vi "Update Objective tree.vi"(7 "Visible Items:Column Headers Visible":bool, 8 "error in (no error)":errorcluster, 9 "Column Header Strings[]":string[](array[string]), 10 "Config cluster IN":T1, 11 "TreeControl in":refnum<vi>) -> (0 "error out":errorcluster)   [LabVIEW 2020]
uses:
  Typedefs/Calibration config.ctl
  Typedefs/Objective Config.ctl
  Typedefs/Prechirper Cal Config.ctl
  Typedefs/PreChirper constants.ctl
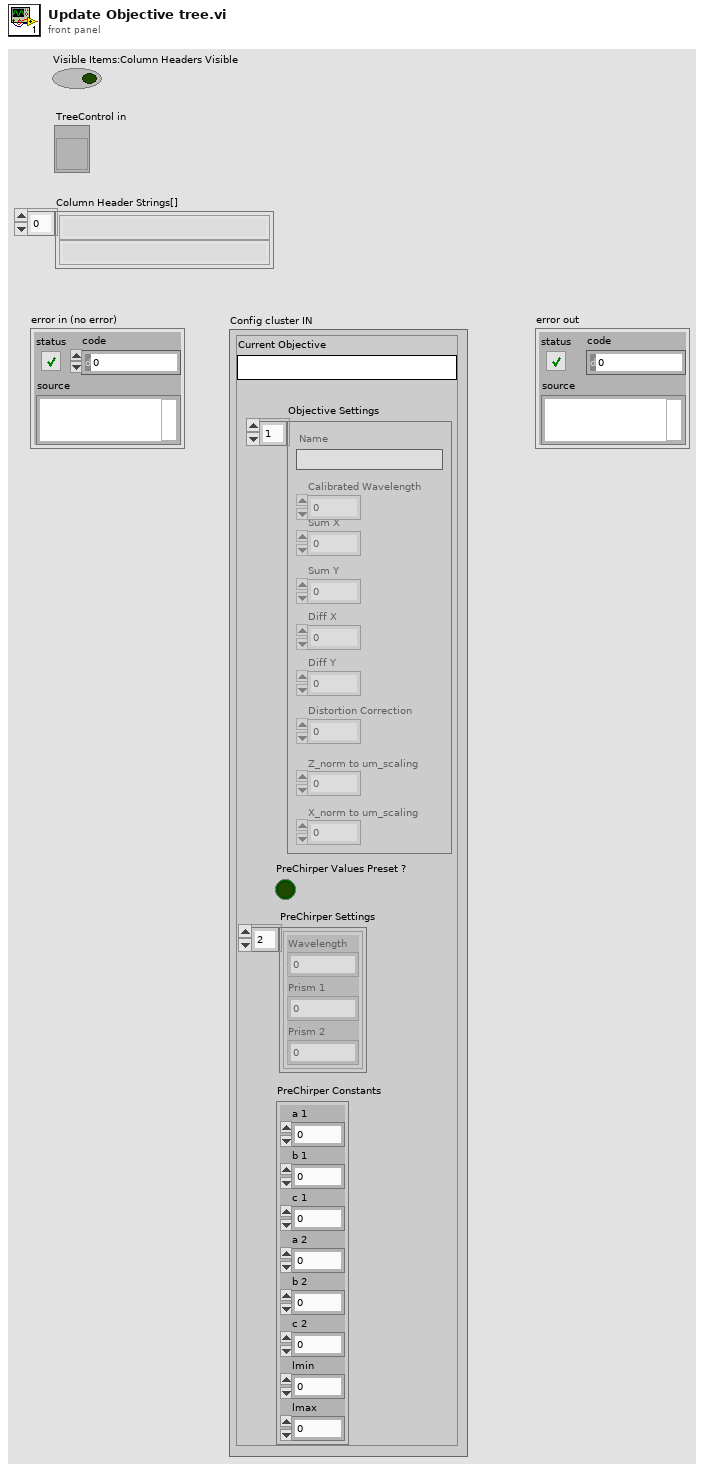
[diagram p1: front panel]
types:
  T1 = typedef "Calibration config.ctl" = cluster{"Current Objective":string, "Objective Settings":T2[], "PreChirper Values Preset ?":bool, "PreChirper Settings":T3[], "PreChirper Constants":T4}
  T2 = typedef "Objective Config.ctl" = cluster{"Name":string, "Sum X":dbl, "Sum Y":dbl, "Diff X":dbl, "Diff Y":dbl, "Distortion Correction":dbl, "Z_norm to um_scaling":dbl, "X_norm to um_scaling":dbl, "Calibrated Wavelength":dbl}
  T3 = typedef "Prechirper Cal Config.ctl" = cluster{"Wavelength":i32, "Prism 1":i32, "Prism 2":i32}
  T4 = typedef "PreChirper constants.ctl" = cluster{"a 1":i32, "b 1":i32, "c 1":i32, "a 2":i32, "b 2":i32, "c 2":i32, "lmin":i32, "lmax":i32}
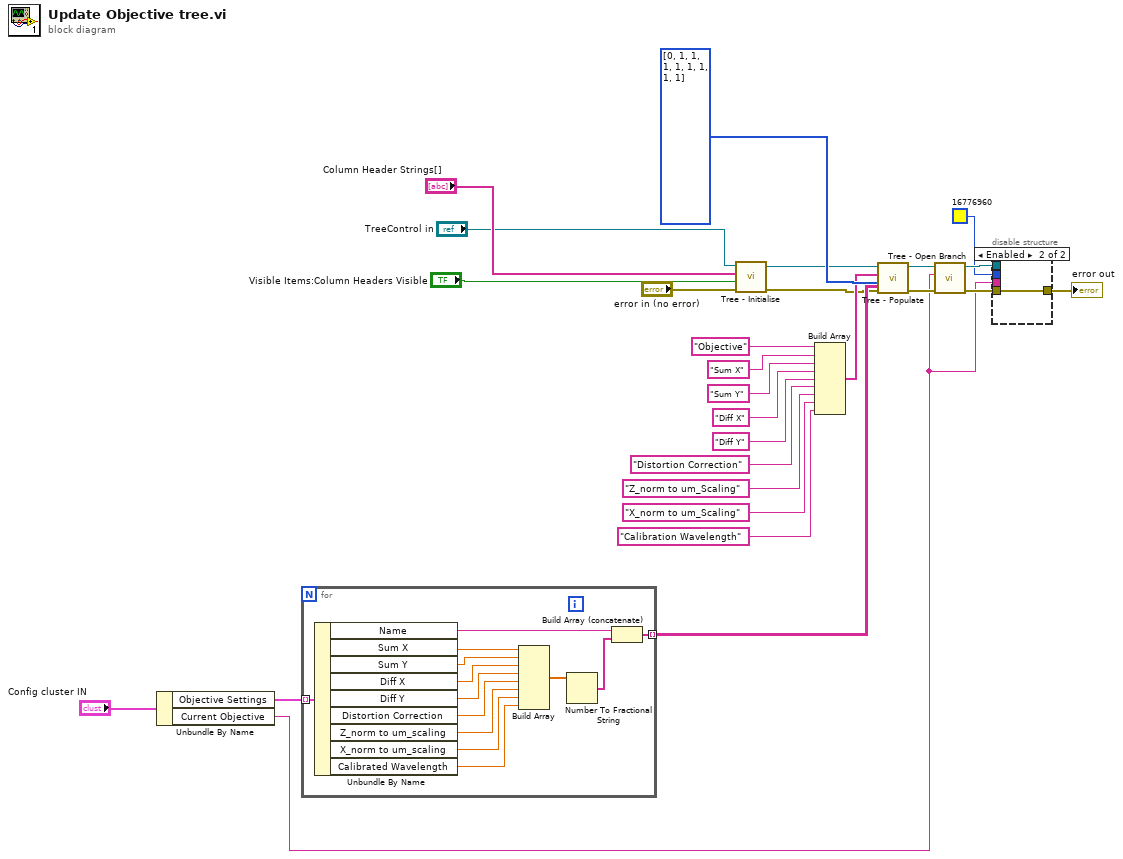
[diagram p0: block diagram]
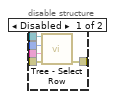
[diagram p2: hidden frame]
diagram:
  n1 = Unbundle By Name("Config cluster IN") -> ("Objective Settings"=w9:T2[], "Current Objective"=w4:string)
  n2 = for {
    tunnel: w9 -> [w40] mode=indexing
    tunnel: [w29] -> w16 mode=indexing
    n3 = Unbundle By Name(w40) -> ("Name"=w28:string, "Sum X"=w39:dbl, "Sum Y"=w38:dbl, "Diff X"=w37:dbl, "Diff Y"=w36:dbl, "Distortion Correction"=w35:dbl, "Z_norm to um_scaling"=w34:dbl, "X_norm to um_scaling"=w33:dbl, "Calibrated Wavelength"=w32:dbl)
    n4 = Build Array(w39, w38, w37, w36, w35, w34, w33, w32) -> (w31:dbl[])
    n5 = Number To Fractional String(number=w31) -> (F-format string=w30:string[])  [unwired: 3 in]
    n6 = Build Array (concatenate)(w28, w30) -> (w29:string[])
  }
  n7 = call "Tree - Initialise.vi"("error in (no error)"="error in (no error)", "Column Headers Visible"="Visible Items:Column Headers Visible", "Column Header Strings[]"="Column Header Strings[]", "TreeControl in"="TreeControl in") -> ("error out"=w10:errorcluster, "TreeControl out"=w11:refnum<vi>)  [unwired: 6 in]
  n8 = Build Array("Objective" ("element"), "Sum X", "Sum Y", "Diff X", "Diff Y", "Distortion Correction", "Z_norm to um_Scaling", "X_norm to um_Scaling", "Calibration Wavelength") -> (w17:string[])
  n9 = call "Tree - Populate.vi"("Item Values"=w16, "error in (no error)"=w10, "Item Indentation"=i32[] [0, 1, 1, 1, 1, 1, 1, 1, 1], "Item Names"=w17, "TreeControl in"=w11) -> ("error out"=w14:errorcluster, "TreeControl out"=w15:refnum<vi>)  [unwired: 5 in]
  n10 = call "Tree - Open Branch.vi"("error in (no error)"=w14, "Tag"=w4, "TreeControl in"=w15) -> ("error out"=w7:errorcluster, "TreeControl out"=w6:refnum<vi>)  [unwired: 7 in]
  n11 = disable-structure shown="Enabled" {
    disable-tunnel: w7 -> [w45 w46]
    disable-tunnel: w6 -> [w44 _]
    disable-tunnel: u32 16776960 ("Color Box") -> [w43 _]
    disable-tunnel: w4 -> [w42 _]
    disable-tunnel: [w41 w46] -> w2
    frame Disabled {
      n12 = call "Tree - Select Row.vi"("error in (no error)"=w45, "Active Cell:String"=w42, "Color Box"=w43, "TreeControl in"=w44) -> ("error out"=w41:errorcluster)  [unwired: 6 in, 1 out]
    }
    frame Enabled {
    }
  }
  "error out" <- w2
